vi "Ping.vi"(8 "error in (no error)":errorcluster, 9 "timeout ms (5000)":i32=5000, 10 "Payload":u8[](array[numeric]), 11 "WebSocket in":refnum<class "WebSocket.lvclass">) -> (0 "error out":errorcluster, 1 "timed out?":bool, 3 "WebSocket out":refnum<class "WebSocket.lvclass">)   [LabVIEW 2021, in "WebSockets.lvlib" / "WebSocket.lvclass"]
doc: "Sends a Ping frame to the connection endpoint. A pong response with the same payload should be received. Can be used as a keep-alive and for determining connection status.\nWebSockets 2.0.1.40\nSam Sharp - MediaMongrels Ltd\nCopyright (c) 2019, MediaMongrels Ltd"
uses:
  WebSocket.lvclass
  Opcodes.ctl
  WebSocket.lvclass/WebSocket.ctl
  DataLengthBytes.vi
  EncodeMaskedBytes.vi
  Socket Write.vi
  Socket Read.vi
  Timing/Calculate Timeout.vi
  Timing/Tick Count with Error Wires.vi
  DecodeMaskedBytes.vi
  Sockets/Socket/Socket.lvclass
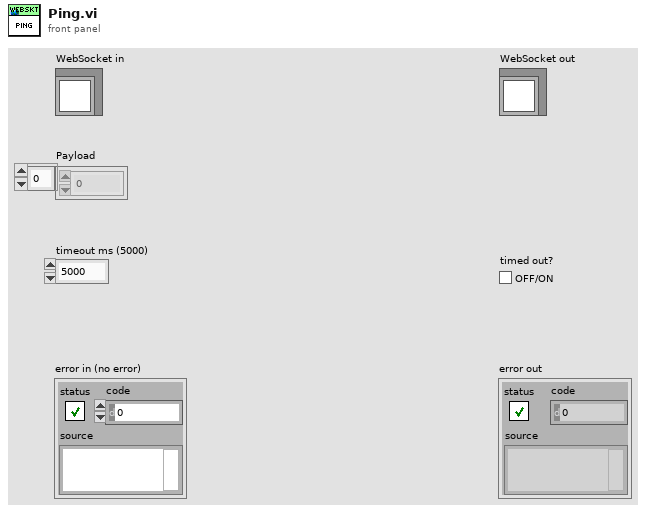
[diagram p1: front panel]
types:
  T1 = typedef "WebSockets.lvlib/WebSocket.lvclass/Opcodes.ctl" = u8
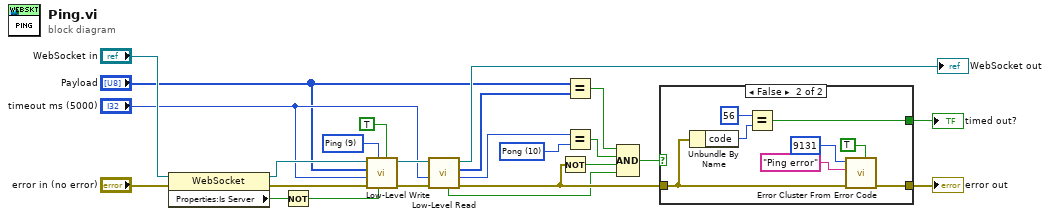
[diagram p0: block diagram]
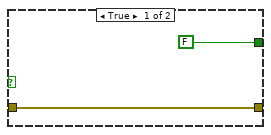
[diagram p2: hidden frame]
diagram:
  w16 = T1 10 items=["Cont. Frame"=0, "Text"=1, "Binary"=2, "Close Frame"=8, "Ping"=9, "Pong"=10] ("Opcode")
  w22 = T1 9 items=["Cont. Frame"=0, "Text"=1, "Binary"=2, "Close Frame"=8, "Ping"=9, "Pong"=10] ("Opcode (Text)")
  n1 = property class="WebSocket"(reference="WebSocket in", error in="error in (no error)") -> (reference out=w19:refnum<class "WebSocket.lvclass">, error out=w21:errorcluster, "Properties:Is Server"=w18:bool)
  n2 = Not(x=w18) -> (.not. x?=w17:bool)
  n3 = call "Low-Level Write.vi"("Finished? (True)"=TRUE, "Mask payload?"=w17, "Opcode (Text)"=w22, "error in (no error)"=w21, "timeout ms (5000)"="timeout ms (5000)", "Data"="Payload", "WebSockets in"=w19) -> ("error out"=w14:errorcluster, "WebSockets out"=w13:refnum<class "WebSocket.lvclass">)  [unwired: 2 in, 1 out]
  n4 = call "Low-Level Read.vi"("error in (no error)"=w14, "timeout ms (5000)"="timeout ms (5000)", "WebSockets in"=w13) -> ("error out"=w5:errorcluster, "Opcode"=w15:T1, "Data"=w10:u8[], "WebSockets out"=→"WebSocket out":refnum<class "WebSocket.lvclass">, "Finished?"=w1:bool)  [unwired: 4 in]
  n5 = Not(x=w5) -> (.not. x?=w6:bool)
  n6 = Equal?(x="Payload", y=w10) -> (x = y?=w8:bool)
  n7 = Equal?(x=w15, y=w16) -> (x = y?=w7:bool)
  n8 = Compound Arithmetic op=AND(w8, w7, w6, w1) -> (w4:bool)
  n9 = case shown="False" w4 {
    tunnel: w5 -> [w26 w30]
    tunnel: [w26 w31] -> w3
    tunnel: [FALSE ("timed out?") w27] -> w2
    frame True {
    }
    frame False {
      n10 = Unbundle By Name(w30) -> ("code"=w29:i32)
      n11 = Equal?(x=56, y=w29) -> (x = y?=w27:bool)
      n12 = call <vilib>:"Error Cluster From Error Code.vi"("is warning? (False)"=TRUE, "error in (no error)"=w30, "error message (\"\")"="Ping error" ("error message (\"\")"), "error code (0)"=9131) -> ("error out"=w31:errorcluster)  [unwired: 5 in]
    }
  }
  "error out" <- w3
  "timed out?" <- w2
